vi "String_Empty buffer define by lenght.vi"(1 "Lenght (255)":i32=255) -> (0 "Empty buffer":string)   [LabVIEW 2020]
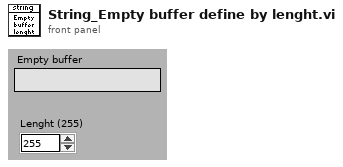
[diagram p1: front panel]
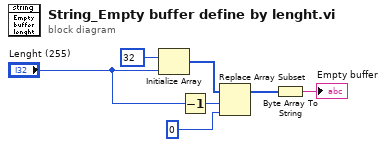
[diagram p0: block diagram]
diagram:
  n1 = Initialize Array(u8 32, "Lenght (255)") -> (w5:u8[])
  n2 = Decrement(x="Lenght (255)") -> (x-1=w2:i32)
  n3 = Replace Array Subset(array=w5, new element=u8 0 ("new element/subarray"), index=w2) -> (w3:u8[])
  n4 = Byte Array To String(unsigned byte array=w3) -> (string=→"Empty buffer":string)
